vi "Set Default Thermocouple Type.vi"(8 "error in (no error)":errorcluster, 10 "Default Thermocouple Type (4: K)":u32(ring)=4 items=["B", "C", "E", "J", "K", "L:Jdin", "N", "R", "S", "T", "U:Tdin", "X", "Y", "Z"], 11 "VISA resource name":refnum<visa-resource-name>) -> (0 "error out":errorcluster, 3 "VISA resource name out":refnum<visa-resource-name>)   [LabVIEW 2011, in "Fluke 5XXX Series Multicalibrators.lvlib"]
doc: "This VI sets the default thermocouple (TC) sensor type, which is saved in the Calibrator non-volatile memory. (While saving configuration data in the non-volatile memory, a period of about 2 seconds, the Calibrator does not respond to remote commands.) The TC type is set to the default at power on and reset.\n\nNote:\n\nThis VI is available only for instrument models 5500A and 5520A."
uses:
  Fluke 5XXX Series Multicalibrators.lvlib
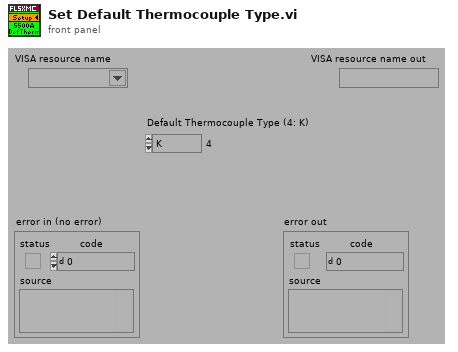
[diagram p1: front panel]
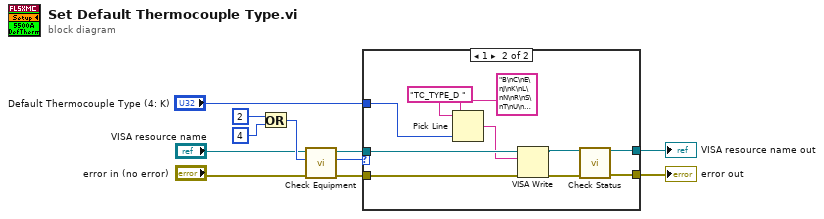
[diagram p0: block diagram]
diagram:
  n1 = Or(x=2 ("Numeric"), y=4 ("Numeric")) -> (x .or. y?=w11:i32)
  n2 = call "Check Equipment.vi"("error in (no error)"="error in (no error)", "Bit Mask"=w11, "VISA resource name"="VISA resource name") -> ("error out"=w10:errorcluster, "Present?"=w9:u32, "VISA resource name out"=w8:refnum<visa-resource-name>)  [unwired: 6 in]
  n3 = case shown="1" w9 {
    tunnel: "Default Thermocouple Type (4: K)" -> [_ w19]
    tunnel: w10 -> [w13 w22]
    tunnel: w8 -> [w12 w21]
    tunnel: [w13 w18] -> w3
    tunnel: [w12 w14] -> w1
    frame 0, Default {
    }
    frame 1 {
      n4 = Pick Line(string ("")="TC_TYPE_D " ("Reset Command"), multi-line string="B\nC\nE\nJ\nK\nL\nN\nR\nS\nT\nU\nX\nY\nZ", line index=w19) -> (output string=w20:string)
      n5 = VISA Write(VISA resource name=w21, write buffer=w20, error in (no error)=w22) -> (VISA resource name out=w16:refnum<visa-resource-name>, error out=w17:errorcluster)  [unwired: 1 out]
      n6 = call "Check Status.vi"("VISA resource name"=w16, "error in (no error)"=w17) -> ("VISA resource name out"=w14:refnum<visa-resource-name>, "error out"=w18:errorcluster)  [unwired: 12 in]
    }
  }
  "VISA resource name out" <- w1
  "error out" <- w3
